vi "niRFUtil MT UTIL Coerror(x) (real array).vi"(1 "x":T1 min=0 max=127 format="%.2f") -> (0 "Coerror(x)":T1 min=0 max=127 format="%.2f")   [LabVIEW 2015, in "niRFUtil.lvlib"]
doc: "Calculates the coerror of X, where X is an array of doubles."
uses:
  niRFUtil.lvlib
  Includes/niRFUtil INC Real Array.ctl
  <vilib>/gmath/NI_Gmath.lvlib
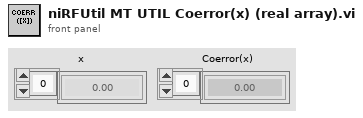
[diagram p1: front panel]
types:
  T1 = typedef "niRFUtil.lvlib/niRFUtil INC Real Array.ctl" = sgl[]
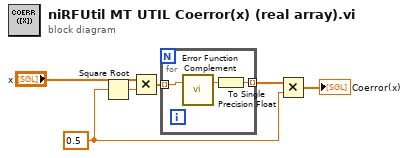
[diagram p0: block diagram]
diagram:
  w1 = sgl 0.5
  n1 = Square Root(x=w1) -> (sqrt(x)=w4:sgl)
  n2 = Multiply(x="x", y=w4) -> (x*y=w5:T1)
  n3 = for {
    tunnel: w5 -> [w9] mode=indexing
    tunnel: [w7] -> w2 mode=indexing
    n4 = call <vilib>:"Error Function Complement.vi"("x"=w9) -> ("1 - erf(x)"=w8:dbl)  [unwired: 2 out]
    n5 = To Single Precision Float(number=w8) -> (single precision float=w7:sgl)
  }
  n6 = Multiply(x=w2, y=w1) -> (x*y=→"Coerror(x)":sgl[])
